vi "Read Control Label.vi"(8 "error in (no error)":errorcluster, 11 "ShortcutMenuSelectionMsg in":refnum<class "ShortcutMenuSelectionMsg.lvclass">) -> (0 "error out":errorcluster, 2 "Control Label":string, 3 "ShortcutMenuSelectionMsg out":refnum<class "ShortcutMenuSelectionMsg.lvclass">)   [LabVIEW 2020, in "ActorEvents.lvlib" / "ShortcutMenuSelectionMsg.lvclass"]
uses:
  <vilib>/gpm_packages/@cs/mva-viewable/Source/ActorEvents/IEventAggregator Messages/ShortcutMenuSelectionMsg/ShortcutMenuSelectionMsg.lvclass
  <vilib>/gpm_packages/@cs/mva-viewable/Source/ActorEvents/IEventAggregator Messages/ShortcutMenuSelectionMsg/ShortcutMenuSelectionMsg.lvclass/ShortcutMenuSelectionMsg.ctl
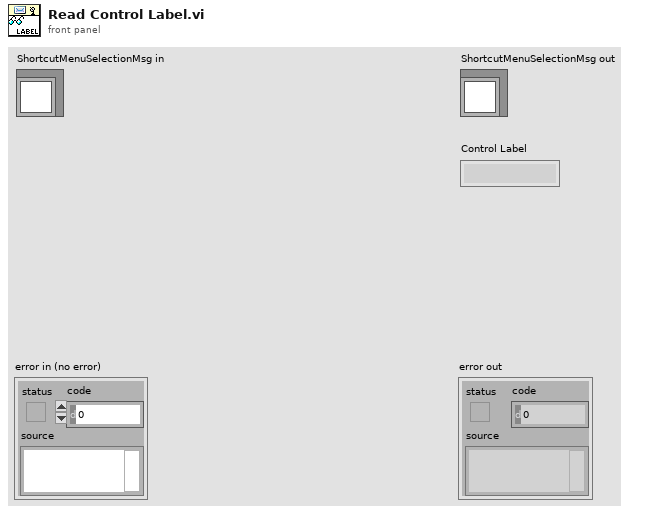
[diagram p1: front panel]
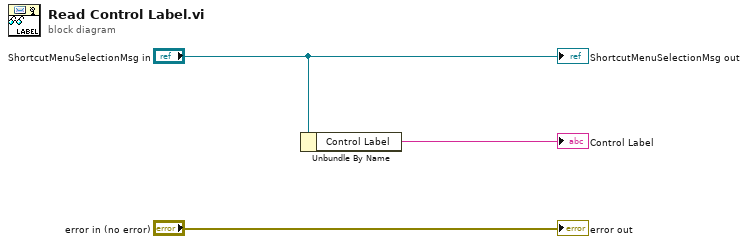
[diagram p0: block diagram]
diagram:
  n1 = Unbundle By Name("ShortcutMenuSelectionMsg in") -> ("Control Label"=→"Control Label":string)
  "error out" <- "error in (no error)"
  "ShortcutMenuSelectionMsg out" <- "ShortcutMenuSelectionMsg in"
